vi "Ticks to Radians.vi"(1 "Ticks":dbl) -> (0 "Radians":dbl)   [LabVIEW 2016]
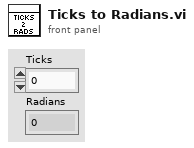
[diagram p1: front panel]
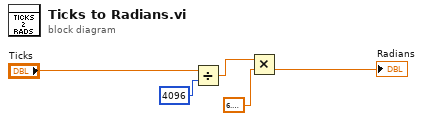
[diagram p0: block diagram]
diagram:
  n1 = Divide(x="Ticks", y=4096) -> (x/y=w4:dbl)
  n2 = Multiply(x=w4, y=6.283185307179586) -> (x*y=→"Radians":dbl)
